vi "command_channel.vi"(0 "command":T1(ring), 1 "channel":string, 2 "data":string, 3 "error in":errorcluster, 5 "connection settings":T2={"Serial port"="COM1", "Network address"="192.168.10.15", "connection method"=enum."PIPE", "Port"=1300, "Pipe name"="\\\\.\\pipe\\channel_system", "Measurement program"="channel_system.exe"}) -> (7 "output":string, 8 "no connection":bool, 9 "error out":errorcluster)   [LabVIEW 2018]
doc: "MeasGUI - Measurement Graphics User Interface\nCopyright (c) 2018 Frans Korhonen\n\nMeasGUI was originally developed at Institute for Atmospheric \nand Earth System Research / Physics, Faculty of Science, \nUniversity of Helsinki, Finland\n\nAssistance, experience and feedback from following persons have been \ncritical in development of MeasGUI: Michel Attoui, Juha Kangasluoma, \nLauri Ahonen, Ella Häkkinen, Markku Kulmala and Tuukka Petäjä.\n\nThis file is part of MeasGUI.\n\nThis Source Code Form is subject to the terms of the Mozilla Public\nLicense, v. 2.0. If a copy of the MPL was not distributed with this\nfile, You can obtain one at http://mozilla.org/MPL/2.0/."
uses:
  <vilib>/Utility/error.llb/DialogType.ctl
  <vilib>/Instr/_visa.llb/VISA Set IO Buffer Mask.ctl
  <vilib>/Instr/_visa.llb/VISA Configure Serial Port (Instr).vi
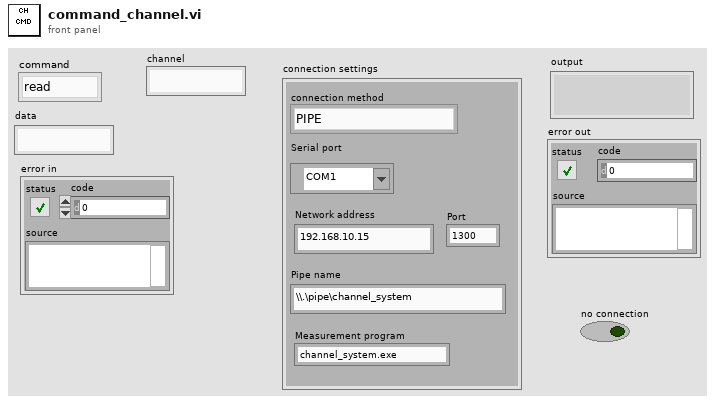
[diagram p1: front panel]
types:
  T1 = enum16{"read", "write", "reset", "conf", "link", "raw communication"}
  T2 = cluster{"Serial port":refnum<visa-resource-name>, "Network address":string, "connection method":enum16{"SERIAL (VISA)", "UDP", "LOCAL", "PIPE", "SERIAL (pipe channel)"}, "Port":u16, "Pipe name":string, "Measurement program":string}
  T3 = enum16{"SERIAL (VISA)", "UDP", "LOCAL", "PIPE", "SERIAL (pipe channel)"}
  T4 = enum16{"start program", "write", "read", "terminate", "clear buffer"}
  T5 = typedef "DialogType.ctl" = u16
  T6 = typedef "VISA Set IO Buffer Mask.ctl" = u16
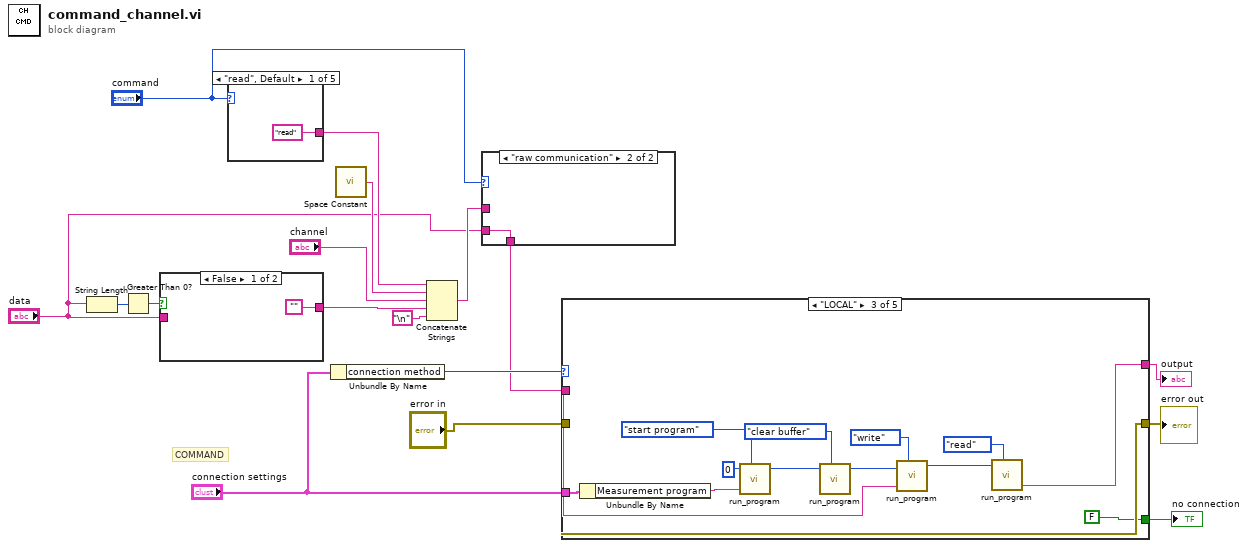
[diagram p0: block diagram]
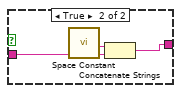
[diagram p3: hidden frame]
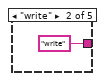
[diagram p4: hidden frame]
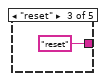
[diagram p5: hidden frame]
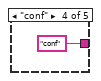
[diagram p6: hidden frame]
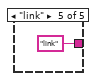
[diagram p7: hidden frame]
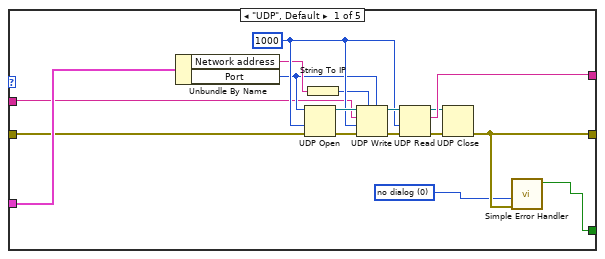
[diagram p8: hidden frame]
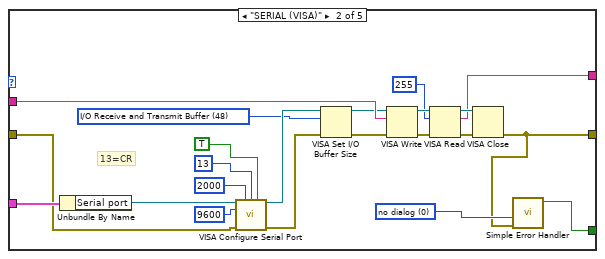
[diagram p9: hidden frame]
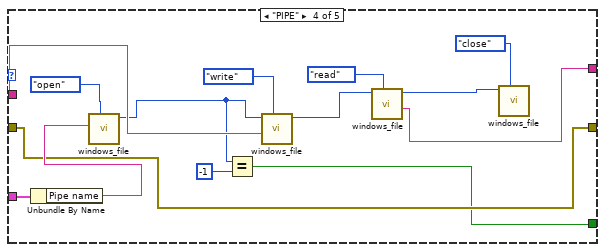
[diagram p10: hidden frame]
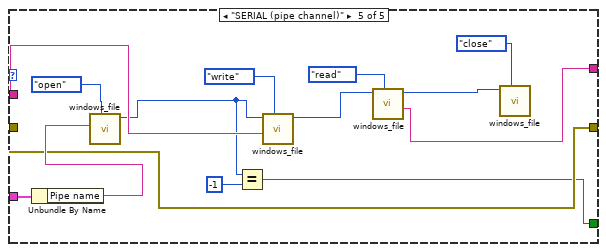
[diagram p11: hidden frame]
diagram:
  # "COMMAND"
  n1 = String Length(string="data") -> (length=w10:i32)
  n2 = Greater Than 0?(x=w10) -> (x > 0?=w9:bool)
  n3 = case shown="False" w9 {
    tunnel: "data" -> [_ w20]
    tunnel: ["" w19] -> w8
    frame False {
    }
    frame True {
      n4 = call <vilib>:"Space Constant.vi"() -> ("String"=w21:string)
      n5 = Concatenate Strings(w21, w20) -> (w19:string)
    }
  }
  n6 = case shown="\"read\", Default" "command" {
    tunnel: ["read" "write" "reset" "conf" "link"] -> w11
    frame "read", Default {
    }
    frame "write" {
    }
    frame "reset" {
    }
    frame "conf" {
    }
    frame "link" {
    }
  }
  n7 = Unbundle By Name("connection settings") -> ("connection method"=w17:T3)
  n8 = call <vilib>:"Space Constant.vi"() -> ("String"=w14:string)
  n9 = Concatenate Strings(w11, w14, "channel", w8, "\n") -> (w5:string)
  n10 = case shown="\"raw communication\"" "command" {
    tunnel: w5 -> [w27 _]
    tunnel: "data" -> [_ w28]
    tunnel: [w27 w28] -> w2
    frame Default {
    }
    frame "raw communication" {
    }
  }
  n11 = case shown="\"LOCAL\"" w17 {
    tunnel: "connection settings" -> [w45 w67 w69 w92 w106]
    tunnel: [w42 w56 w74 w87 w101] -> w15
    tunnel: w2 -> [w33 w59 w72 w90 w104]
    tunnel: [w31 w47 w73 w85 w99] -> w12
    tunnel: "error in" -> [w32 w51 w73 w85 w99]
    tunnel: [w29 w46 FALSE w82 w96] -> w1
    frame "UDP", Default {
      w30 = T5 0 items=["no dialog", "OK message", "continue or stop message", "OK message + warnings", "continue/stop + warnings"] ("type of dialog (OK msg:1)")
      w41 = 1000 ("timeout ms (25000)")
      n12 = Unbundle By Name(w45) -> ("Network address"=w39:string, "Port"=w38:u16)
      n13 = UDP Open(8:w32, 9:w41, 11:w38) -> (port=w43:refnum<k16>, 0:w34:errorcluster)  [unwired: 2 in, 1 out]
      n14 = String To IP(1:w39) -> (0:w40:u32)
      n15 = UDP Write(address=w40, port or service name=w38, connection ID=w43, data in=w33, 8:w34, 9:w41) -> (error out=w35:errorcluster, 3:w44:refnum<k16>)
      n16 = UDP Read(connection ID=w44, timeout ms (25000)=w41, 8:w35) -> (data out=w42:string, error out=w36:errorcluster, 3:w37:refnum<k16>)  [unwired: 1 in, 2 out]
      n17 = UDP Close(connection ID=w37, 8:w36) -> (error out=w31:errorcluster)  [unwired: 1 out]
      n18 = call <vilib>:"Simple Error Handler.vi"("type of dialog (OK msg:1)"=w30, "error in (no error)"=w31) -> ("error?"=w29:bool)  [unwired: 3 in, 4 out]
    }
    frame "SERIAL (VISA)" {
      w48 = T5 0 items=["no dialog", "OK message", "continue or stop message", "OK message + warnings", "continue/stop + warnings"] ("type of dialog (OK msg:1)")
      w58 = T6 48 items=["I/O Receive Buffer"=16, "I/O Transmit Buffer"=32, "I/O Receive and Transmit Buffer"=48] ("Mask")
      # "13=CR"
      n19 = Unbundle By Name(w67) -> ("Serial port"=w62:refnum<visa-resource-name>)
      n20 = call-poly "VISA Configure Serial Port"("VISA resource name"=w62, "timeout (10sec)"=u32 2000, "termination char\n(0xA = '\\n' = LF)"=u8 13 ("termination char\n(0xA = '\\n' = LF)"), "Enable Termination\nChar (T)"=TRUE ("Enable Termination\nChar (T)"), "baud rate (9600)"=u32 9600, "error in (no error)"=w51) -> ("VISA resource name out"=w60:refnum<visa-resource-name>, "error out"=w61:errorcluster)  [unwired: 8 in]
      n21 = VISA Set I/O Buffer Size(VISA resource name=w60, mask (16)=w58, error in (no error)=w61) -> (VISA resource name out=w49:refnum<visa-resource-name>, error out=w50:errorcluster)  [unwired: 1 in]
      n22 = VISA Write(VISA resource name=w49, write buffer=w59, error in (no error)=w50) -> (VISA resource name out=w55:refnum<visa-resource-name>, error out=w54:errorcluster)  [unwired: 1 out]
      n23 = VISA Read(VISA resource name=w55, byte count=u32 255, error in (no error)=w54) -> (VISA resource name out=w57:refnum<visa-resource-name>, read buffer=w56:string, error out=w52:errorcluster)  [unwired: 1 out]
      n24 = VISA Close(VISA resource name=w57, error in (no error)=w52) -> (error out=w47:errorcluster)
      n25 = call <vilib>:"Simple Error Handler.vi"("type of dialog (OK msg:1)"=w48, "error in (no error)"=w47) -> ("error?"=w46:bool)  [unwired: 3 in, 4 out]
    }
    frame "LOCAL" {
      n26 = Unbundle By Name(w69) -> ("Measurement program"=w68:string)
      n27 = call "run_program.vi"("program id in"=u32 0, "operation"=T4."start program", "data in"=w68) -> ("program id out"=w77:u32)  [unwired: 2 in, 2 out]
      n28 = call "run_program.vi"("program id in"=w77, "operation"=T4."clear buffer") -> ("program id out"=w76:u32)  [unwired: 3 in, 2 out]
      n29 = call "run_program.vi"("program id in"=w76, "operation"=T4."write", "data in"=w72) -> ("program id out"=w75:u32)  [unwired: 2 in, 2 out]
      n30 = call "run_program.vi"("program id in"=w75, "operation"=T4."read") -> ("data out"=w74:string)  [unwired: 3 in, 2 out]
    }
    frame "PIPE" {
      n31 = Unbundle By Name(w92) -> ("Pipe name"=w86:string)
      n32 = call "windows_file.vi"("operation"=enum16{"open", "close", "read", "write"}."open", "FileName"=w86) -> ("handle_out"=w84:i32)  [unwired: 8 in, 1 out]
      n33 = Equal?(x=w84, y=-1) -> (x = y?=w82:bool)
      n34 = call "windows_file.vi"("operation"=enum16{"open", "close", "read", "write"}."write", "string_in"=w90, "handle_in"=w84) -> ("handle_out"=w89:i32)  [unwired: 7 in, 1 out]
      n35 = call "windows_file.vi"("operation"=enum16{"open", "close", "read", "write"}."read", "handle_in"=w89) -> ("string_out"=w87:string, "handle_out"=w88:i32)  [unwired: 8 in]
      n36 = call "windows_file.vi"("operation"=enum16{"open", "close", "read", "write"}."close", "handle_in"=w88) -> ()  [unwired: 8 in, 2 out]
    }
    frame "SERIAL (pipe channel)" {
      n37 = Unbundle By Name(w106) -> ("Pipe name"=w100:string)
      n38 = call "windows_file.vi"("operation"=enum16{"open", "close", "read", "write"}."open", "FileName"=w100) -> ("handle_out"=w97:i32)  [unwired: 8 in, 1 out]
      n39 = Equal?(x=w97, y=-1) -> (x = y?=w96:bool)
      n40 = call "windows_file.vi"("operation"=enum16{"open", "close", "read", "write"}."write", "string_in"=w104, "handle_in"=w97) -> ("handle_out"=w103:i32)  [unwired: 7 in, 1 out]
      n41 = call "windows_file.vi"("operation"=enum16{"open", "close", "read", "write"}."read", "handle_in"=w103) -> ("string_out"=w101:string, "handle_out"=w102:i32)  [unwired: 8 in]
      n42 = call "windows_file.vi"("operation"=enum16{"open", "close", "read", "write"}."close", "handle_in"=w102) -> ()  [unwired: 8 in, 2 out]
    }
  }
  "output" <- w15
  "error out" <- w12
  "no connection" <- w1
